vi "Update Buffers.vi"(8 "error in (no error)":errorcluster, 11 "HistorianCharting in":refnum<class "HistorianCharting.lvclass">) -> (0 "error out":errorcluster, 3 "HistorianCharting out":refnum<class "HistorianCharting.lvclass">)   [LabVIEW 2020, in "VolatusGUIElements.lvlib" / "HistorianCharting.lvclass"]
uses:
  HistorianCharting.lvclass
  HistorianCharting.lvclass/HistorianCharting.ctl
  Volatus/VolatusAPI/VolatusAPI.lvclass
  Volatus/MessageQ/MessageQ.lvclass
  VolatusHistorian/Group Buffer DBL/Group Buffer DBL.lvclass
  Buffer Info.ctl
  e09d2c7e-15e9-49d1-ab6b-5da3d5d60274.vi
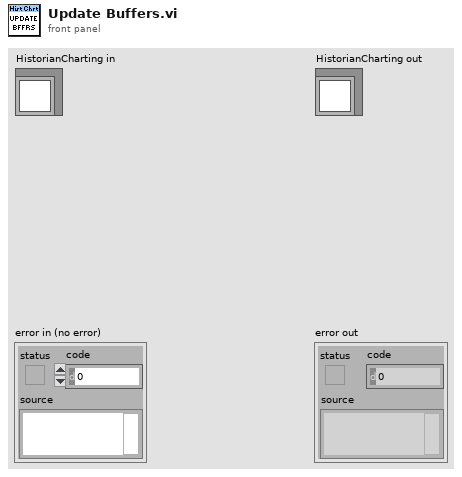
[diagram p1: front panel]
types:
  T1 = typedef "VolatusGUIElements.lvlib/HistorianCharting.lvclass/Buffer Info.ctl" = cluster{"Buffer":refnum<class "Group Buffer DBL.lvclass">, "Channels":string[], "Plot Indices":i32[]}
  T2 = typedef "VolatusGUI.lvlib/Historian Charting Manager.lvclass/Plot Config.ctl" = cluster{"Channel":string, "Visible":bool, "Color":u32, "Scale":T3}
  T3 = typedef "VolatusGUI.lvlib/Historian Charting Manager.lvclass/Scale.ctl" = enum16{"Left", "Right"}
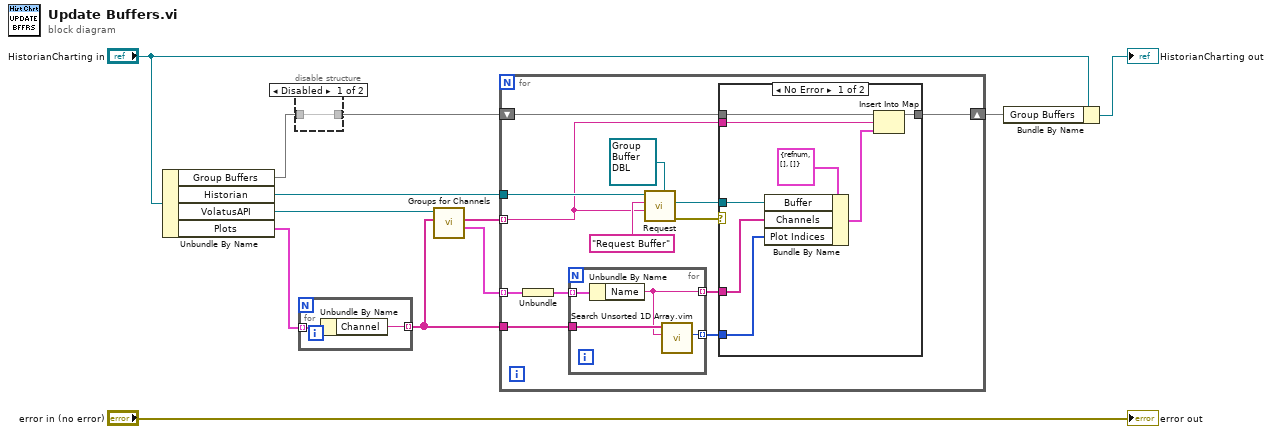
[diagram p0: block diagram]
diagram:
  n1 = Unbundle By Name("HistorianCharting in") -> ("Group Buffers"=w10:map{string, T1}, "Historian"=w6:refnum<class "MessageQ.lvclass">, "VolatusAPI"=w8:refnum<class "VolatusAPI.lvclass">, "Plots"=w9:T2[])
  n2 = disable-structure shown="Disabled" {
    disable-tunnel: w10 -> [w13 _]
    disable-tunnel: [w13 _] -> w7
    frame Disabled {
    }
    frame Enabled {
    }
  }
  n3 = for {
    tunnel: w9 -> [w15] mode=indexing
    tunnel: [w14] -> w3 mode=indexing
    n4 = Unbundle By Name(w15) -> ("Channel"=w14:string)
  }
  n5 = call "Groups for Channels.vi"("Channels"=w3, "VolatusAPI in"=w8) -> ("Channels per Group"=w4:cluster{cluster{"Index":i32, "Name":string}[]}[], "Groups"=w5:string[])  [unwired: 6 in, 2 out]
  n6 = for {
    tunnel: w6 -> [w28]
    tunnel: w5 -> [w16] mode=indexing
    shift-right: [w19] -> w1
    shift-left: w7 -> [w25]
    tunnel: w4 -> [w24] mode=indexing
    tunnel: w3 -> [w20]
    n7 = Unbundle(w24) -> (w23:cluster{"Index":i32, "Name":string}[])
    n8 = for {
      tunnel: w23 -> [w41] mode=indexing
      tunnel: [w39] -> w21 mode=indexing
      tunnel: w20 -> [w40]
      tunnel: [w38] -> w18 mode=indexing
      n9 = Unbundle By Name(w41) -> ("Name"=w39:string)
      n10 = call "Search Unsorted 1D Array.vim"("element"=w39, "unsorted 1D array"=w40) -> ("index of element"=w38:i32)  [unwired: 9 in]
    }
    n11 = call "Request.vi"("Response Type (None)"=refnum<class "Group Buffer DBL.lvclass"> refnum ("VolatusHistorian.lvlib:Group Buffer DBL.lvclass"), "Data"=w16, "ID"="Request Buffer", "MessageQ in"=w28) -> ("error out"=w17:errorcluster, "Response"=w22:refnum<class "Group Buffer DBL.lvclass">)  [unwired: 5 in, 1 out]
    n12 = case shown="No Error" w17 {
      tunnel: w25 -> [w36 w37]
      tunnel: w22 -> [w33 _]
      tunnel: w21 -> [w32 _]
      tunnel: [w31 w37] -> w19
      tunnel: w18 -> [w30 _]
      tunnel: w16 -> [w29 _]
      frame No Error {
        n13 = Bundle By Name(cluster=T1 {"Buffer"=refnum, "Channels"=[], "Plot Indices"=[]} ("value"), "Buffer"=w33, "Channels"=w32, "Plot Indices"=w30) -> (w34:T1)
        n14 = Insert Into Map(map in=w36, key=w29, value=w34) -> (map out=w31:map{string, T1})  [unwired: 2 out]
      }
      frame Error {
      }
    }
  }
  n15 = Bundle By Name(cluster="HistorianCharting in", "Group Buffers"=w1) -> (→"HistorianCharting out":refnum<class "HistorianCharting.lvclass">)
  "error out" <- "error in (no error)"
